vi "Ask_488_on.vi"(8 "error in":errorcluster, 11 "VISA resource name":refnum<visa-resource-name>) -> (0 "error out":errorcluster, 2 "488 On":bool, 3 "VISA resource name out":refnum<visa-resource-name>)   [LabVIEW 2015]
uses:
  <vilib>/Instr/_visa.llb/VISA Configure Serial Port (Instr).vi
panel:
  out "debug":string
  out "Serial Settings:Number of Bytes at Serial Port":u32
  out "read buffer":string
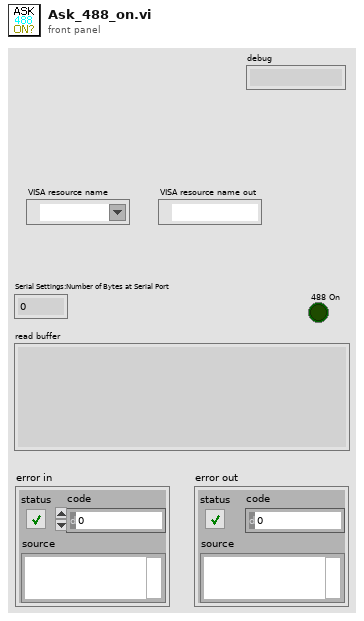
[diagram p1: front panel]
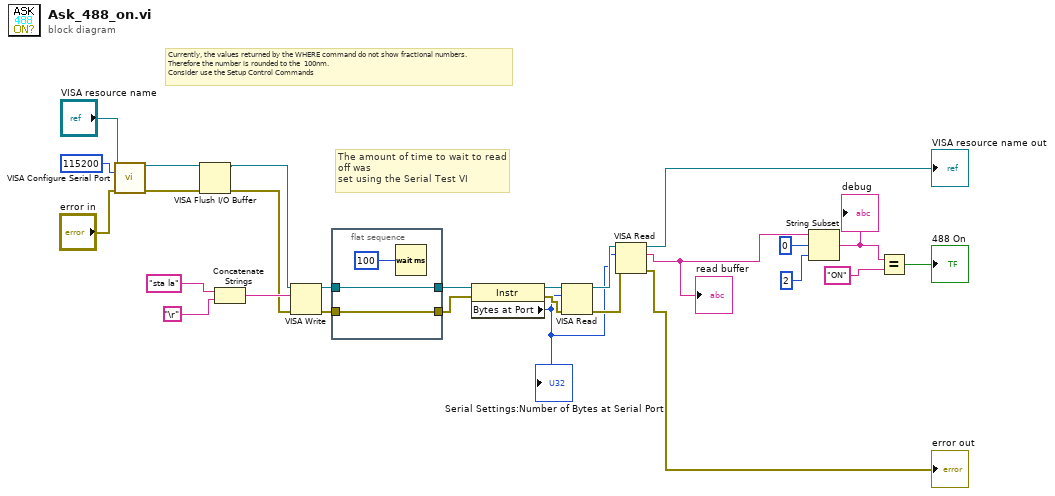
[diagram p0: block diagram]
diagram:
  # "Currently, the values returned by the WHERE command do not show fractional numbers.\nTherefore the number is rounded to the  100nm. \nConsider use the Setup Control Commands"
  # "The amount of time to wait to read off was \nset using the Serial Test VI"
  n1 = call-poly "VISA Configure Serial Port"("VISA resource name"="VISA resource name", "baud rate (9600)"=u32 115200, "error in (no error)"="error in") -> ("VISA resource name out"=w3:refnum<visa-resource-name>, "error out"=w4:errorcluster)  [unwired: 11 in]
  n2 = VISA Flush I/O Buffer(VISA resource name=w3, error in (no error)=w4) -> (VISA resource name out=w2:refnum<visa-resource-name>, error out=w1:errorcluster)  [unwired: 1 in]
  n3 = Concatenate Strings("sta la" ("string"), "\r") -> (w21:string)
  n4 = VISA Write(VISA resource name=w2, write buffer=w21, error in (no error)=w1) -> (VISA resource name out=w25:refnum<visa-resource-name>, error out=w23:errorcluster)  [unwired: 1 out]
  n5 = flat-sequence {
    tunnel: [w30] -> w26
    tunnel: w25 -> [w30]
    tunnel: [w28] -> w24
    tunnel: w23 -> [w28]
    frame #0 {
      n6 = Wait (ms)(milliseconds to wait=u32 100) -> ()  [unwired: 1 out]
    }
  }
  n7 = property class="Instr"(reference=w26, error in=w24) -> (reference out=w27:refnum<visa-resource-name>, error out=w22:errorcluster, "Bytes at Port"=w9:u32)
  "Serial Settings:Number of Bytes at Serial Port" <- w9
  n8 = VISA Read(VISA resource name=w27, byte count=w9, error in (no error)=w22) -> (VISA resource name out=w12:refnum<visa-resource-name>, error out=w13:errorcluster)  [unwired: 2 out]
  n9 = VISA Read(VISA resource name=w12, byte count=w9, error in (no error)=w13) -> (VISA resource name out=→"VISA resource name out":refnum<visa-resource-name>, read buffer=w8:string, error out=→"error out":errorcluster)  [unwired: 1 out]
  "read buffer" <- w8
  n10 = String Subset(string=w8, offset (0)=0, length (rest)=2 ("length (rest)")) -> (substring=w15:string)
  "debug" <- w15
  n11 = Equal?(x=w15, y="ON" ("regular expression")) -> (x = y?=→"488 On":bool)
